vi "get result counts.vi"(11 "test cases":T1[](array[typedef])) -> (0 "passed":i32, 1 "error":i32, 2 "skipped":i32, 3 "failures":i32)   [LabVIEW 2013]
uses:
  <vilib>/utf/common/utf_test_result_testcase.ctl
  <vilib>/utf/common/utf_test_result.ctl
  <vilib>/utf/common/utf_test_result_troll_new.ctl
  <vilib>/utf/common/utf_vector_result.ctl
  <vilib>/utf/common/utf_test_result_failure.ctl
  <vilib>/utf/common/utf_test_comparison_operators.ctl
  <vilib>/utf/common/utf_vi_tag.ctl
  <vilib>/utf/common/utf_test_result_input_data.ctl
  <vilib>/utf/common/utf_code_coverage.ctl
  <vilib>/utf/NI_UnitTestFramework.lvlib
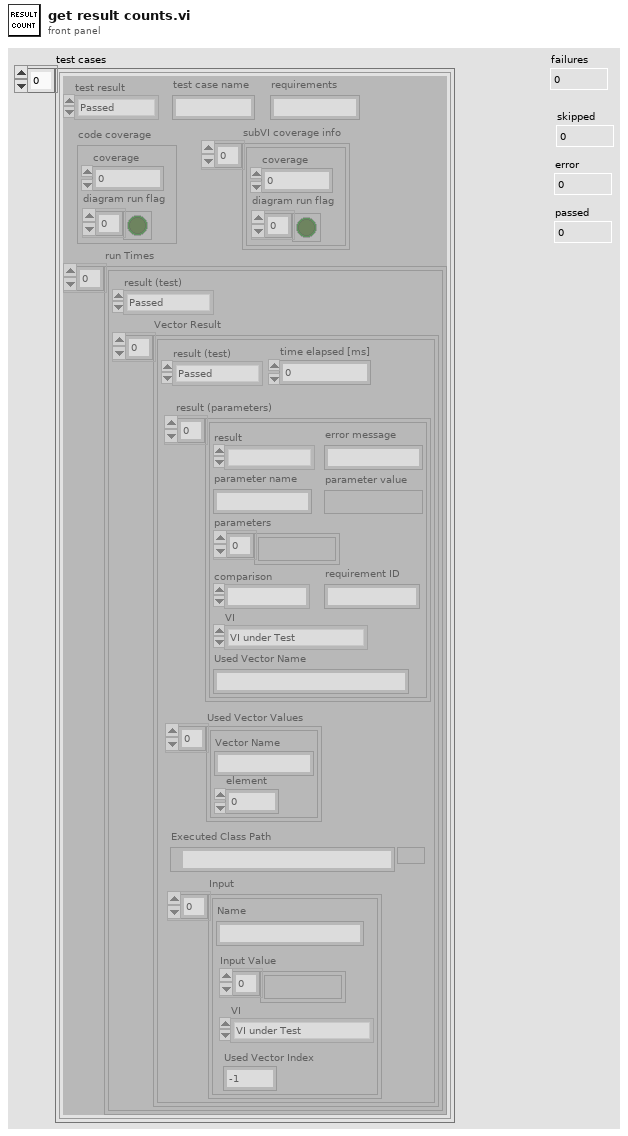
[diagram p1: front panel]
types:
  T1 = typedef "NI_UnitTestFramework.lvlib/utf_test_result_testcase.ctl" = cluster{"test result":T2, "run Times":T3[], "test case name":string, "requirements":string, "code coverage":T9, "subVI coverage info":T9[]}
  T2 = typedef "NI_UnitTestFramework.lvlib/utf_test_result.ctl" = enum16{"Passed", "Failed", "Error", "Skipped", "Not Processed"}
  T3 = typedef "NI_UnitTestFramework.lvlib/utf_test_result_troll_new.ctl" = cluster{"result (test)":T2, "Vector Result":T4[]}
  T4 = typedef "NI_UnitTestFramework.lvlib/utf_vector_result.ctl" = cluster{"time elapsed [ms]":u32, "result (test)":T2, "result (parameters)":T5[], "Used Vector Values":cluster{"Vector Name":string, "element":i32}[], "Executed Class Path":path, "Input":T8[]}
  T5 = typedef "NI_UnitTestFramework.lvlib/utf_test_result_failure.ctl" = cluster{"result":T2, "error message":string, "parameter name":string, "parameter value":variant, "parameters":variant[], "comparison":T6, "requirement ID":string, "VI":T7, "Used Vector Name":string}
  T6 = typedef "NI_UnitTestFramework.lvlib/utf_test_comparison_operators.ctl" = enum16{"=", "!=", ">", ">=", "<", "<=", "range", "symmetric tolerance", "asymmetric tolerance", "string contains", "string not contain", "array size", "string length", "array range", "by element", "array range (limit array)", "user-defined", "array contains", "array not contain", "vector length", "= (elm)", "!= (elm)", "= (case insensitive)", "!= (case insensitive)"}
  T7 = typedef "NI_UnitTestFramework.lvlib/utf_vi_tag.ctl" = enum16{"Setup VI", "VI under Test", "Teardown VI"}
  T8 = typedef "NI_UnitTestFramework.lvlib/utf_test_result_input_data.ctl" = cluster{"Name":string, "Input Value":variant[], "VI":T7, "Used Vector Index":i32}
  T9 = typedef "NI_UnitTestFramework.lvlib/utf_code_coverage.ctl" = cluster{"coverage":dbl, "diagram run flag":bool[]}
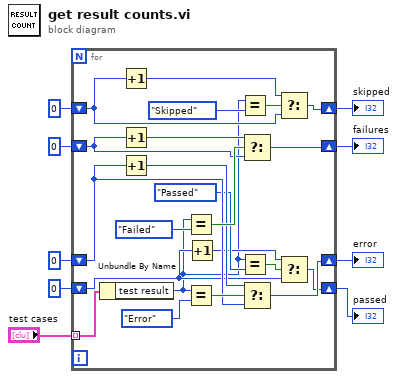
[diagram p0: block diagram]
diagram:
  n1 = for {
    tunnel: "test cases" -> [w31] mode=indexing
    shift-right: [w26] -> w7
    shift-left: 0 -> [w27]
    shift-right: [w25] -> w6
    shift-left: 0 -> [w24]
    shift-right: [w16] -> w3
    shift-left: 0 -> [w17]
    shift-right: [w12] -> w1
    shift-left: 0 -> [w13]
    n2 = Unbundle By Name(w31) -> ("test result"=w11:T2)
    n3 = Increment(x=w24) -> (x+1=w23:i32)
    n4 = Increment(x=w27) -> (x+1=w28:i32)
    n5 = Increment(x=w17) -> (x+1=w18:i32)
    n6 = Equal?(x=w11, y=utf_test_result."Failed") -> (x = y?=w29:bool)
    n7 = Equal?(x=w11, y=utf_test_result."Error") -> (x = y?=w19:bool)
    n8 = Increment(x=w13) -> (x+1=w14:i32)
    n9 = Equal?(x=w11, y=utf_test_result."Skipped") -> (x = y?=w22:bool)
    n10 = Equal?(x=w11, y=utf_test_result."Passed") -> (x = y?=w10:bool)
    n11 = Select(t=w28, s=w29, f=w27) -> (s? t:f=w26:i32)
    n12 = Select(t=w18, s=w19, f=w17) -> (s? t:f=w16:i32)
    n13 = Select(t=w23, s=w22, f=w24) -> (s? t:f=w25:i32)
    n14 = Select(t=w14, s=w10, f=w13) -> (s? t:f=w12:i32)
  }
  "failures" <- w7
  "skipped" <- w6
  "error" <- w3
  "passed" <- w1
